vi "TKPS252XG Configure OVP-OCP24.vi"(0 "VISA session":refnum<visa-resource-name>, 1 "ocp (off:f)":bool, 2 "ovp limit":dbl=7.0 min=0.0 max=38.5 step=0.5 format="%.2f", 3 "error in (no error)":errorcluster, 4 "channel (ch1:0)":u16(ring) items=["channel 1", "channel 2", "channel 3"]) -> (5 "dup VISA session":refnum<visa-resource-name>, 6 "error out":errorcluster)   [LabVIEW 2024]
doc: "This vi sets the OVP limit and turns the over current protection on or off."
panel:
  # "on\n\noff"
  # "----->"
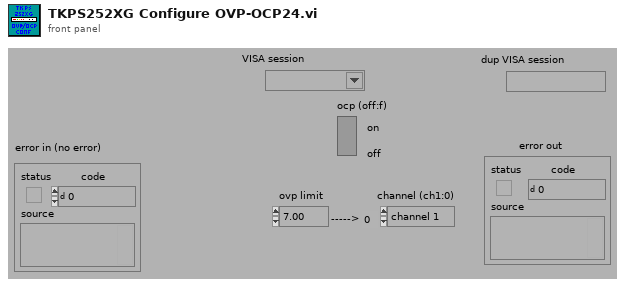
[diagram p1: front panel]
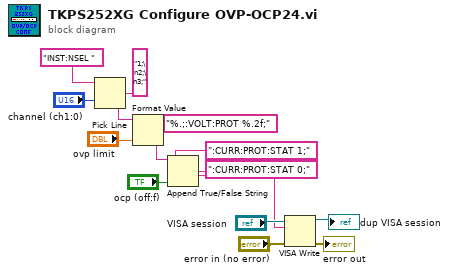
[diagram p0: block diagram]
diagram:
  n1 = Pick Line(string ("")="INST:NSEL " ("VI name"), multi-line string="1;\n2;\n3;" ("VI name"), line index="channel (ch1:0)") -> (output string=w5:string)
  n2 = Format Value(string ("")=w5, format string="%.;:VOLT:PROT %.2f;", value (0)="ovp limit") -> (output string=w2:string)
  n3 = Append True/False String(1:"ocp (off:f)", 2:":CURR:PROT:STAT 0;", 3:":CURR:PROT:STAT 1;", 4:w2) -> (0:w1:string)
  n4 = VISA Write(VISA resource name="VISA session", write buffer=w1, error in (no error)="error in (no error)") -> (VISA resource name out=→"dup VISA session":refnum<visa-resource-name>, error out=→"error out":errorcluster)  [unwired: 1 out]
